vi "measurment_load_cell.vi"() -> ()   [LabVIEW 2024]
uses:
  <vilib>/xnet/xnet.llb/XNET Read (Signal Single-point).vi
  <vilib>/xnet/xnet.llb/XNET Create Session (Signal Input Single-point).vi
panel:
  out "Waveform Chart 4":dbl(graph)
  out "Waveform Chart 3":dbl(graph)
  out "Waveform Chart 2":dbl(graph)
  out "Waveform Chart":dbl(graph)
  out "x+y":dbl[](array[numeric])
  in  "stop":bool
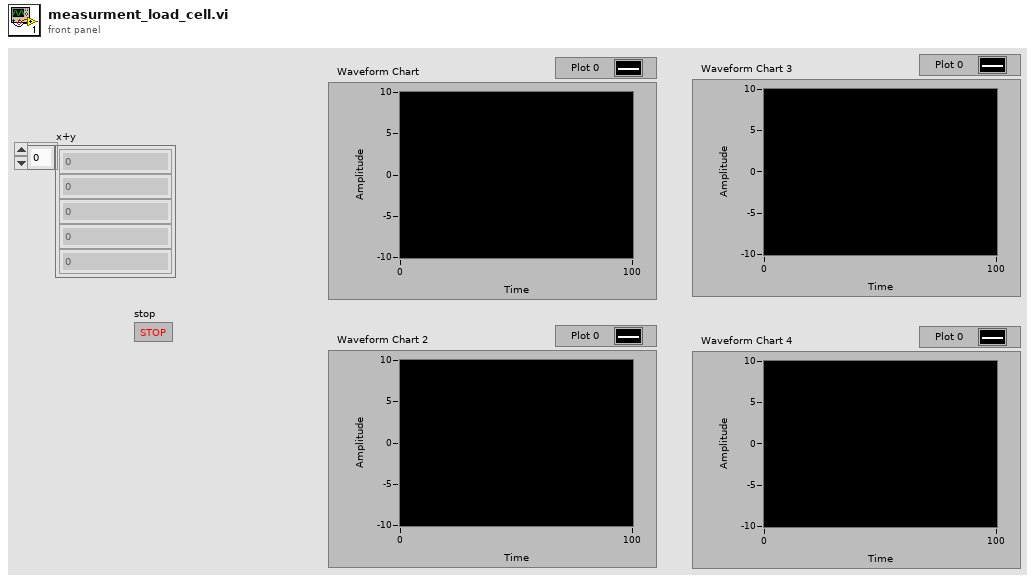
[diagram p1: front panel]
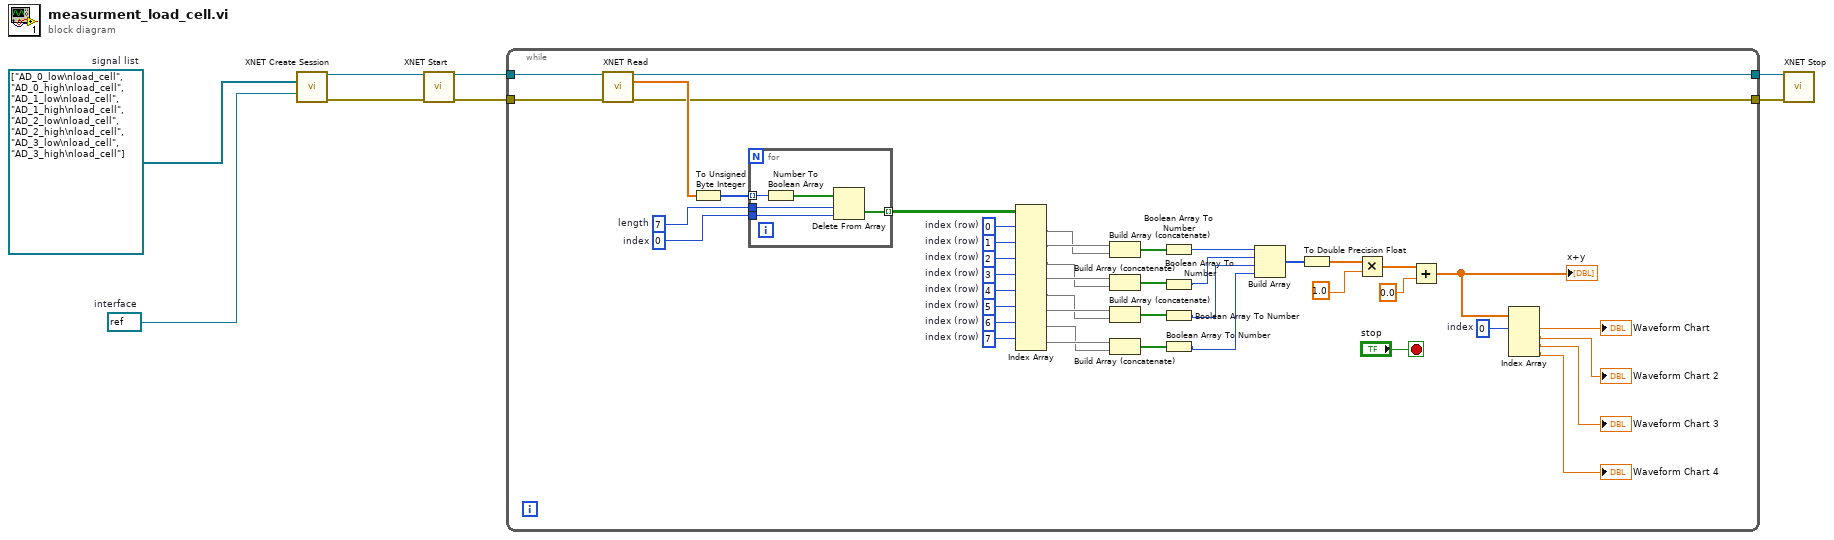
[diagram p0: block diagram]
diagram:
  w7 = refnum<k21> refnum  # interface
  w8 = refnum<k21>[] ["AD_0_low\nload_cell", "AD_0_high\nload_cell", "AD_1_low\nload_cell", "AD_1_high\nload_cell", "AD_2_low\nload_cell", "AD_2_high\nload_cell", "AD_3_low\nload_cell", "AD_3_high\nload_cell"]  # signal list
  n1 = call-poly <vilib>:"XNET Create Session.vi"("signal list"=w8, "interface"=w7) -> ("session out"=w6:refnum<k21>, "error out"=w5:errorcluster)  [unwired: 12 in]
  n2 = call <vilib>:"XNET Start.vi"("session in"=w6, "error in (no error)"=w5) -> ("session out"=w4:refnum<k21>, "error out"=w3:errorcluster)  [unwired: 12 in]
  n3 = while {
    tunnel: w4 -> [w53]
    tunnel: w3 -> [w52]
    tunnel: [w16] -> w2
    tunnel: [w15] -> w1
    stop <- "stop" stop-if-true
    w13 = 0  # index
    w39 = 7  # index (row)
    w40 = 6  # index (row)
    w41 = 5  # index (row)
    w42 = 4  # index (row)
    w43 = 3  # index (row)
    w44 = 2  # index (row)
    w45 = 1  # index (row)
    w46 = 0  # index (row)
    w48 = 7  # length
    w49 = 0  # index
    n4 = call-poly <vilib>:"XNET Read.vi"("session in"=w53, "error in (no error)"=w52) -> ("session out"=w16:refnum<k21>, "data"=w51:dbl[], "error out"=w15:errorcluster)  [unwired: 11 in]
    n5 = To Unsigned Byte Integer(number=w51) -> (unsigned 8bit integer=w50:u8[])
    n6 = for {
      tunnel: [w54] -> w47 mode=indexing
      tunnel: w50 -> [w58] mode=indexing
      tunnel: w49 -> [w56]
      tunnel: w48 -> [w55]
      n7 = Number To Boolean Array(number=w58) -> (Boolean array=w57:bool[])
      n8 = Delete From Array(array=w57, length=w55, index=w56) -> (deleted portion=w54:bool[])  [unwired: 1 out]
    }
    n9 = Index Array "Index Array"(array=w47, index (row) #1=w46, index (row) #2=w45, index (row) #3=w44, index (row) #4=w43, index (row) #5=w42, index (row) #6=w41, index (row) #7=w40, index (row) #8=w39) -> (element #1=w37:bool[], element #2=w38:bool[], element #3=w35:bool[], element #4=w36:bool[], element #5=w33:bool[], element #6=w34:bool[], element #7=w31:bool[], element #8=w32:bool[])  [unwired: 8 in]
    n10 = Build Array (concatenate)(w38, w37) -> (w30:bool[])
    n11 = Build Array (concatenate)(w36, w35) -> (w29:bool[])
    n12 = Build Array (concatenate)(w34, w33) -> (w28:bool[])
    n13 = Build Array (concatenate)(w32, w31) -> (w27:bool[])
    n14 = Boolean Array To Number(Boolean array=w30) -> (number=w26:u32)
    n15 = Boolean Array To Number(Boolean array=w29) -> (number=w25:u32)
    n16 = Boolean Array To Number(Boolean array=w28) -> (number=w24:u32)
    n17 = Boolean Array To Number(Boolean array=w27) -> (number=w23:u32)
    n18 = Build Array(w26, w25, w24, w23) -> (w22:u32[])
    n19 = To Double Precision Float(number=w22) -> (double precision float=w21:dbl[])
    n20 = Multiply(x=w21, y=1.0) -> (x*y=w20:dbl[])
    n21 = Add(x=w20, y=0.0) -> (x+y=w14:dbl[])
    "x+y" <- w14
    n22 = Index Array(array=w14, index #1=w13) -> (element #1=→"Waveform Chart":dbl, element #2=→"Waveform Chart 2":dbl, element #3=→"Waveform Chart 3":dbl, element #4=→"Waveform Chart 4":dbl)  [unwired: 3 in]
  }
  n23 = call <vilib>:"XNET Stop.vi"("session in"=w2, "error in (no error)"=w1) -> ()  [unwired: 12 in, 2 out]
